vi "Default Log File.vi"() -> (1 "Default Log File Name":path)   [LabVIEW 2020, in "RxnRover.lvlib" / "logging.lvlib"]
doc: "Returns a log file name of the form \"<date>_<time>_log.txt\" where the date and time correspond to the first call to this function."
uses:
  logging.lvlib
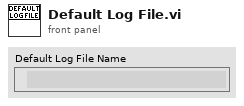
[diagram p1: front panel]
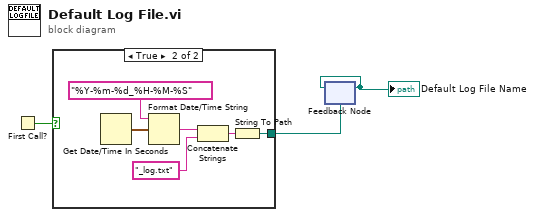
[diagram p0: block diagram]
diagram:
  n1 = First Call?() -> (First Call?: T/F=w3:bool)
  n2 = case shown="True" w3 {
    tunnel: [_ w9] -> w2
    frame False {
    }
    frame True {
      n3 = Get Date/Time In Seconds() -> (seconds since 1Jan1904=w4:timestamp)
      n4 = Format Date/Time String(time format string (%c)="%Y-%m-%d_%H-%M-%S", seconds (now)=w4) -> (date/time string=w6:string)  [unwired: 1 in]
      n5 = Concatenate Strings(w6, "_log.txt" ("time format string (%c)")) -> (w8:string)
      n6 = String To Path(string=w8) -> (path=w9:path)
    }
  }
  n7 = feedback #1(w2) -> (w1:path)
  "Default Log File Name" <- w1
  n8 = feedback-in #1(w1) -> ()
